vi "prep cal image.vi"(0 "Raw cal image":dbl[][](array[numeric]), 1 "LOW bandpass\n(mode)":sgl format="%.2f", 2 "HIGH bandpass\n(mode)":sgl format="%.2f", 3 "forget radius":i32, 4 "# of points (cross size)":i32=128) -> (5 "r-shifted corkscrew cal":cdb[][](array[numeric]), 6 "r shifted cal ampl":dbl[][](array[numeric]), 7 "r shifted cal real":dbl[][](array[numeric]))   [LabVIEW 2014]
uses:
  <vilib>/Analysis/2dsp.llb/Real FFT.vi
  <vilib>/Analysis/2dsp.llb/Inverse Complex FFT.vi
  <vilib>/Analysis/NI_AALPro.lvlib
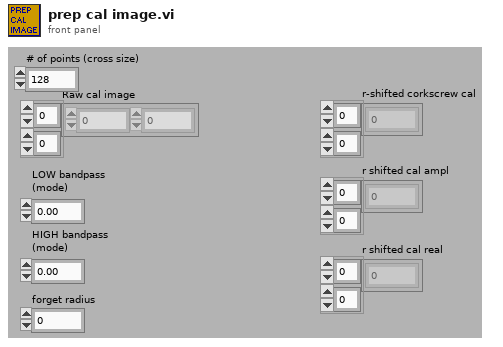
[diagram p1: front panel]
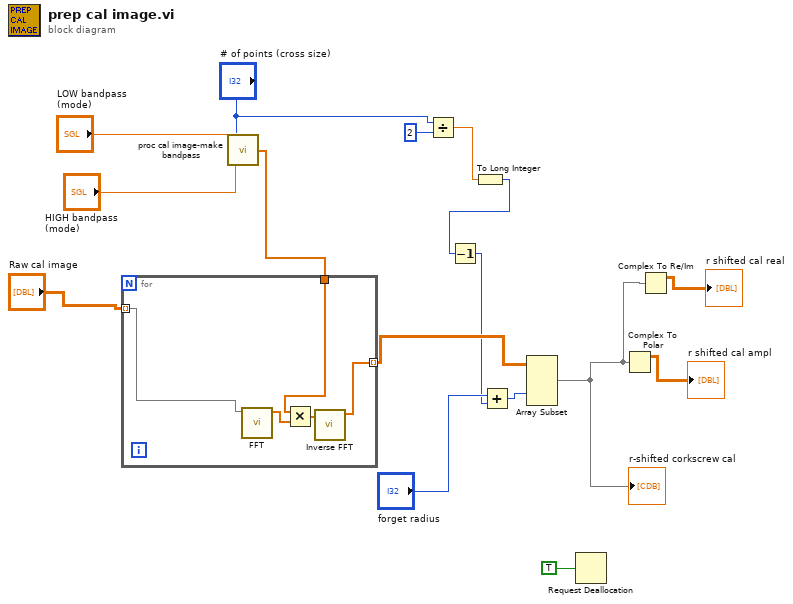
[diagram p0: block diagram]
diagram:
  n1 = call "proc cal image-make bandpass.vi"("HIGH bandpass\n(mode)"="HIGH bandpass\n(mode)", "LOW bandpass\n(mode)"="LOW bandpass\n(mode)", "# of points (cross size)"="# of points (cross size)") -> ("Cosine bandpass"=w12:sgl[])
  n2 = for {
    tunnel: "Raw cal image" -> [w17] mode=indexing
    tunnel: w12 -> [w19]
    tunnel: [w18] -> w10 mode=indexing
    n3 = call-poly <vilib>:"FFT.vi"("X"=w17) -> ("FFT {X}"=w21:cdb[])  [unwired: 2 in, 8 out]
    n4 = Multiply(x=w19, y=w21) -> (x*y=w20:cdb[])
    n5 = call-poly <vilib>:"Inverse FFT.vi"("FFT {X}"=w20) -> ("X"=w18:cdb[])  [unwired: 1 in, 9 out]
  }
  n6 = Divide(x="# of points (cross size)", y=2) -> (x/y=w3:dbl)
  n7 = To Long Integer(number=w3) -> (32bit integer=w2:i32)
  n8 = Decrement(x=w2) -> (x-1=w1:i32)
  n9 = Add(x="forget radius", y=w1) -> (x+y=w16:i32)
  n10 = Array Subset(array=w10, index (col)=w16) -> (w9:cdb[][])  [unwired: 3 in]
  "r-shifted corkscrew cal" <- w9
  n11 = Request Deallocation(TRUE ("flag")) -> ()
  n12 = Complex To Polar(r * e^(i*theta)=w9) -> (r=→"r shifted cal ampl":dbl[][])  [unwired: 1 out]
  n13 = Complex To Re/Im(x + iy=w9) -> (x=→"r shifted cal real":dbl[][])  [unwired: 1 out]
